vi "Line Send Message.vi"(8 "error in":errorcluster, 10 "Message":string, 11 "Token":string) -> (0 "error out":errorcluster, 3 "Reply":string)   [LabVIEW 2020]
uses:
  <vilib>/httpClient/POSTBuffer.vi
  <vilib>/httpClient/LabVIEWHTTPClient.lvlib
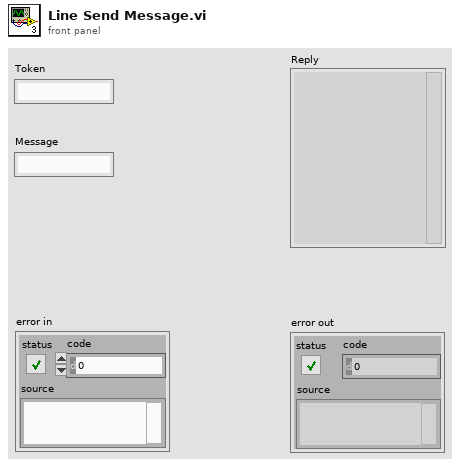
[diagram p1: front panel]
types:
  T1 = typedef "LabVIEWHTTPClient.lvlib/ClientHandle.ctl" = refnum<k1>
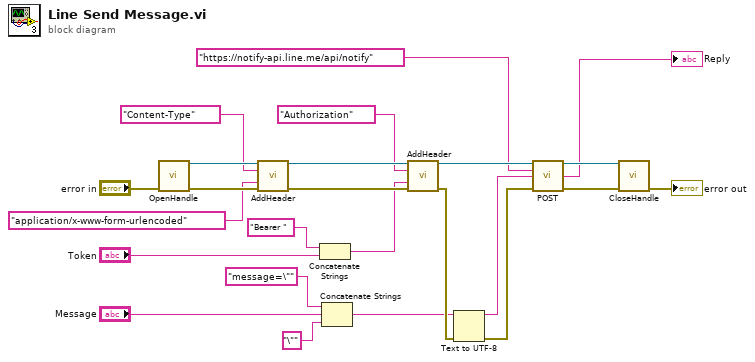
[diagram p0: block diagram]
diagram:
  n1 = call <vilib>:"OpenHandle.vi"("error in (no error)"="error in") -> ("client handle out"=w24:T1, "error out"=w23:errorcluster)  [unwired: 13 in]
  n2 = call <vilib>:"AddHeader.vi"("client handle"=w24, "header"="Content-Type", "value"="application/x-www-form-urlencoded", "error in (no error)"=w23) -> ("client handle out"=w20:T1, "error out"=w19:errorcluster)  [unwired: 10 in]
  n3 = Concatenate Strings("Bearer " ("string"), "Token") -> (w15:string)
  n4 = Concatenate Strings("message=\"" ("string"), "Message", "\"" ("string")) -> (w11:string)
  n5 = call <vilib>:"AddHeader.vi"("client handle"=w20, "header"="Authorization", "value"=w15, "error in (no error)"=w19) -> ("client handle out"=w13:T1, "error out"=w14:errorcluster)  [unwired: 10 in]
  n6 = Text to UTF-8(8:w14, 11:w11) -> (0:w7:errorcluster, 3:w9:string)  [unwired: 1 in]
  n7 = call-poly <vilib>:"POST.vi"("client handle"=w13, "url"="https://notify-api.line.me/api/notify", "buffer"=w9, "error in (no error)"=w7) -> ("client handle out"=w6:T1, "body"=→"Reply":string, "error out"=w5:errorcluster)  [unwired: 8 in, 1 out]
  n8 = call <vilib>:"CloseHandle.vi"("client handle"=w6, "error in (no error)"=w5) -> ("error out"=→"error out":errorcluster)  [unwired: 13 in]
